vi "BRig_RT__Case_Exp__State_initTrial2__v11.vi"(0 "input_dataCurrent":u16[](array[numeric]), 1 "input_dataTrial":u16[][](array[numeric]), 3 "input_dataExp":u16[](array[numeric]), 6 "input_dataBlock":u16[][](array[numeric]), 8 "input_dataLC":u16[](array[numeric])) -> (7 "output_L_Wrong_Laser_l2":bool, 9 "output_L_Wrong_Event_l2":bool, 10 "output_L_Power_l1":dbl, 11 "output_L_Reward_Laser_l2":bool, 12 "output_L_Power_l2":dbl, 13 "output_L_Reward_Event_l2":bool, 14 "output_dataCurrent":u16[](array[numeric]), 15 "output_dataTrial":u16[][](array[numeric]), 16 "output_L_Reward_Event_l1":bool, 17 "output_L_Reward_Laser_l1":bool, 18 "output_L_Wrong_Event_l1":bool, 19 "output_L_Wrong_Laser_l1":bool)   [LabVIEW 2014]
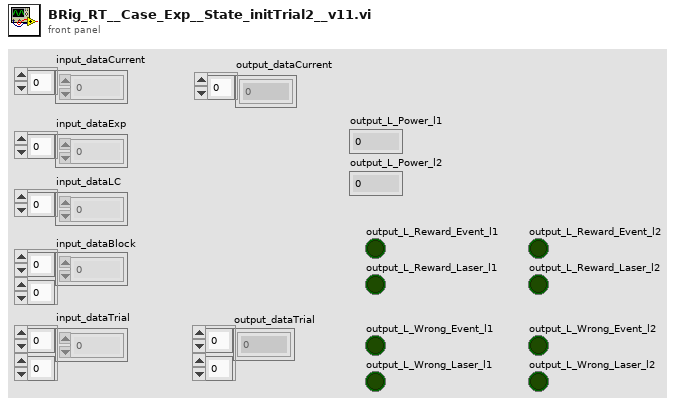
[diagram p1: front panel]
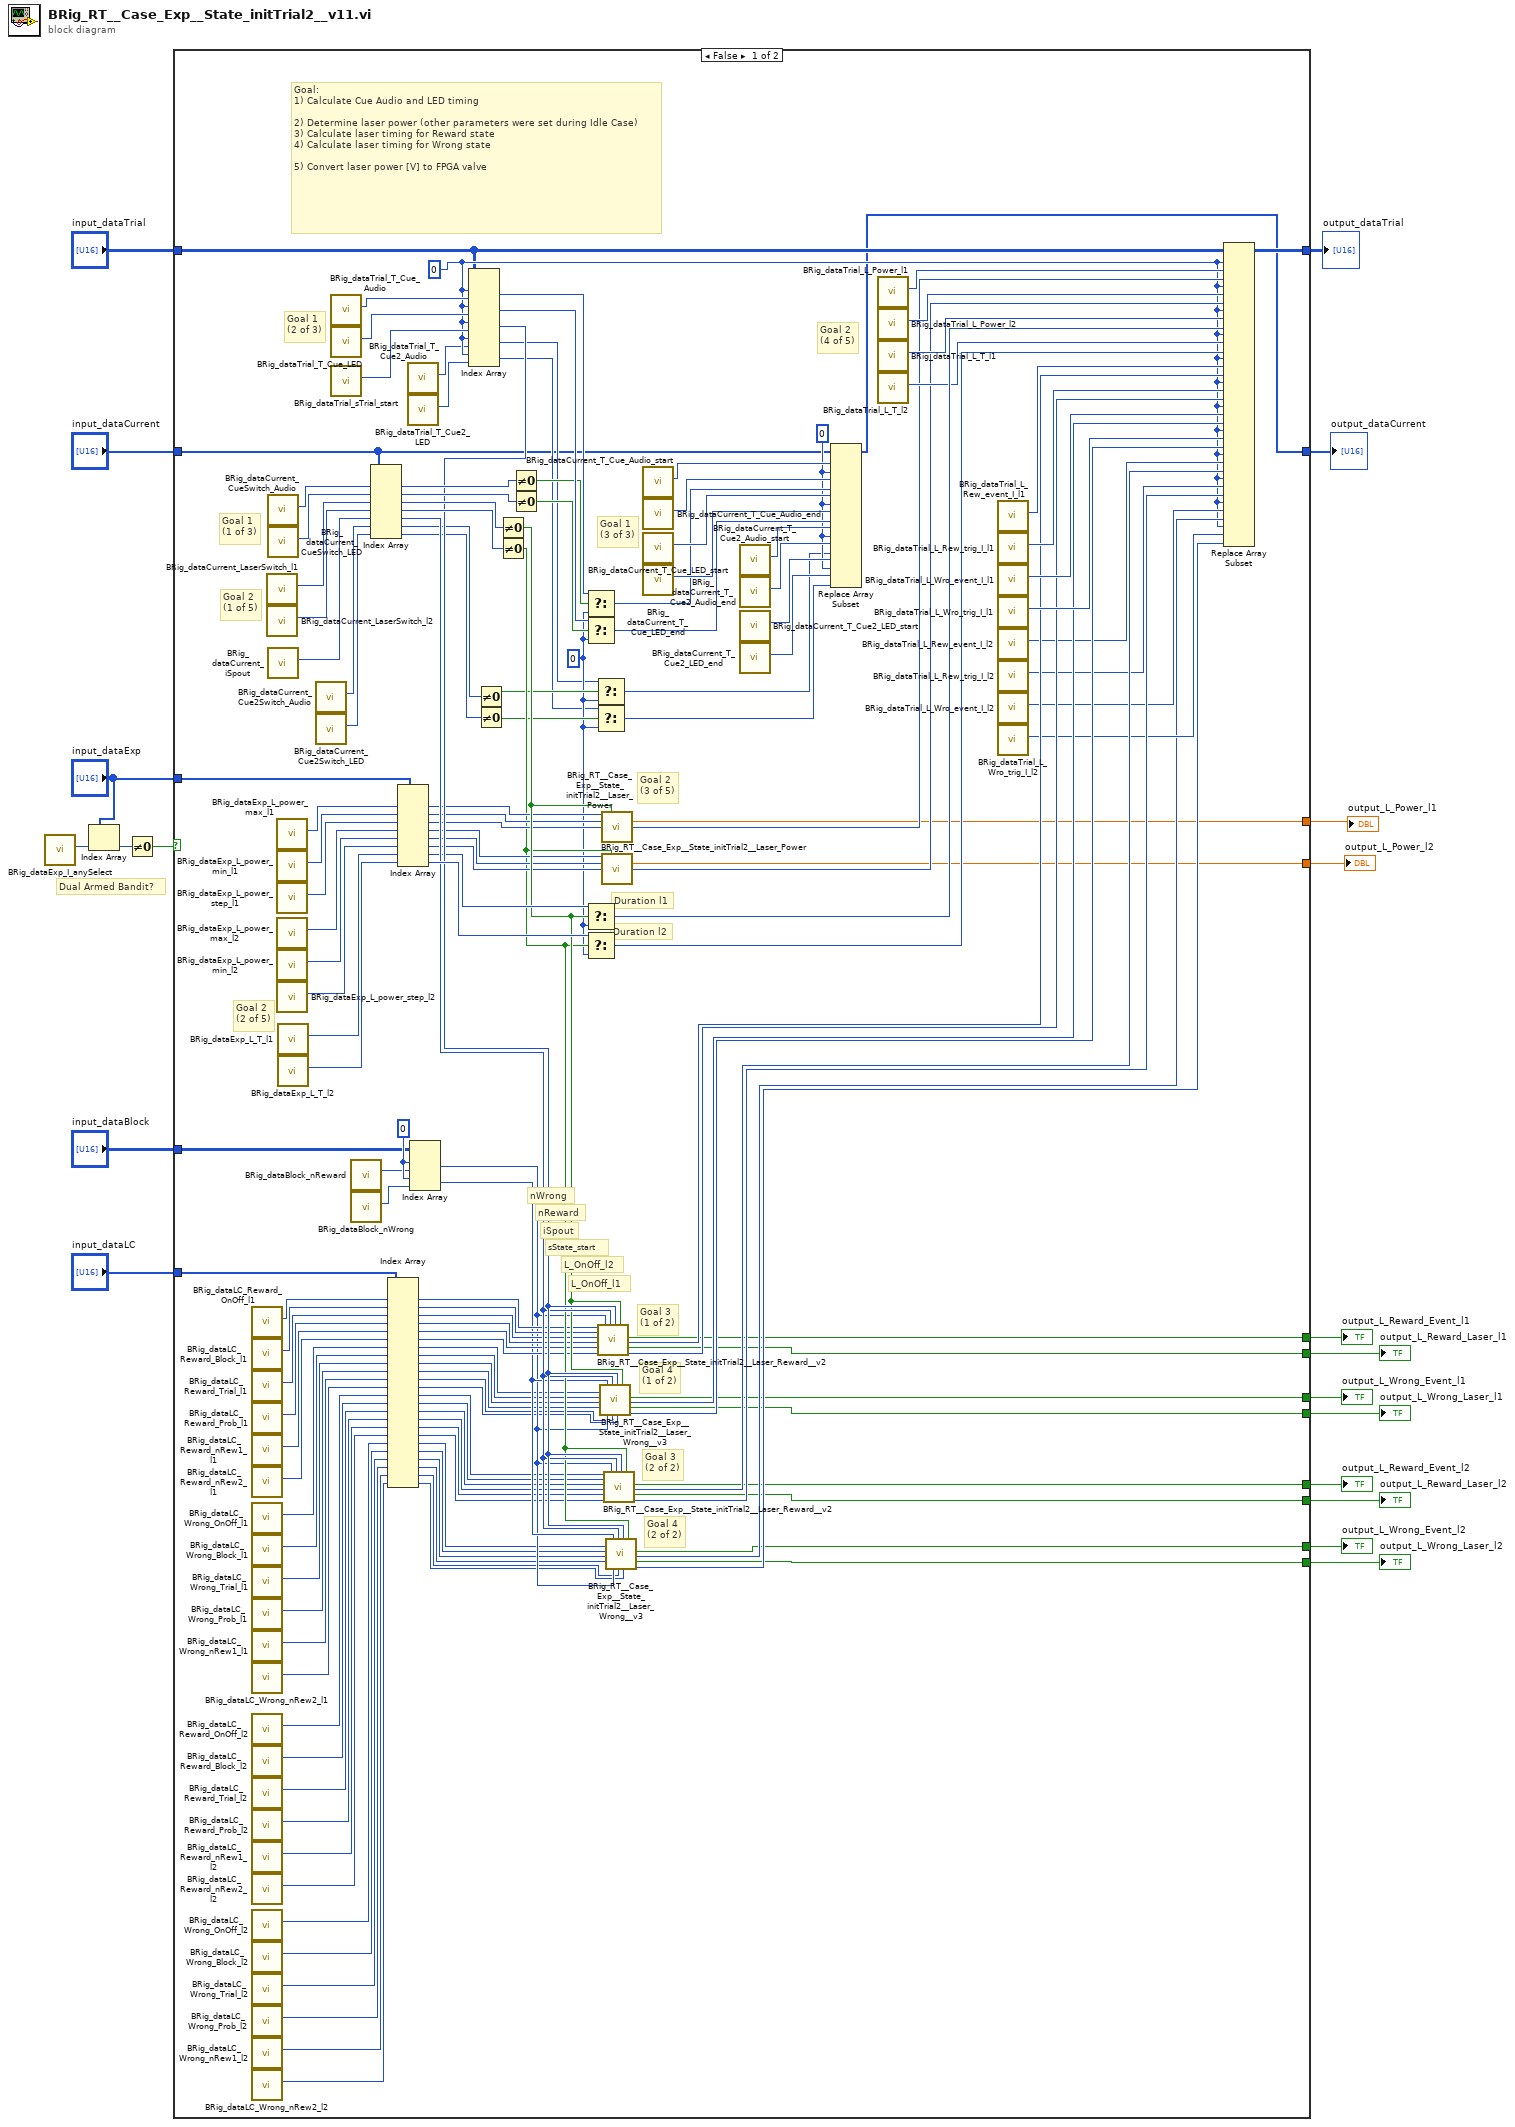
[diagram p0: block diagram]
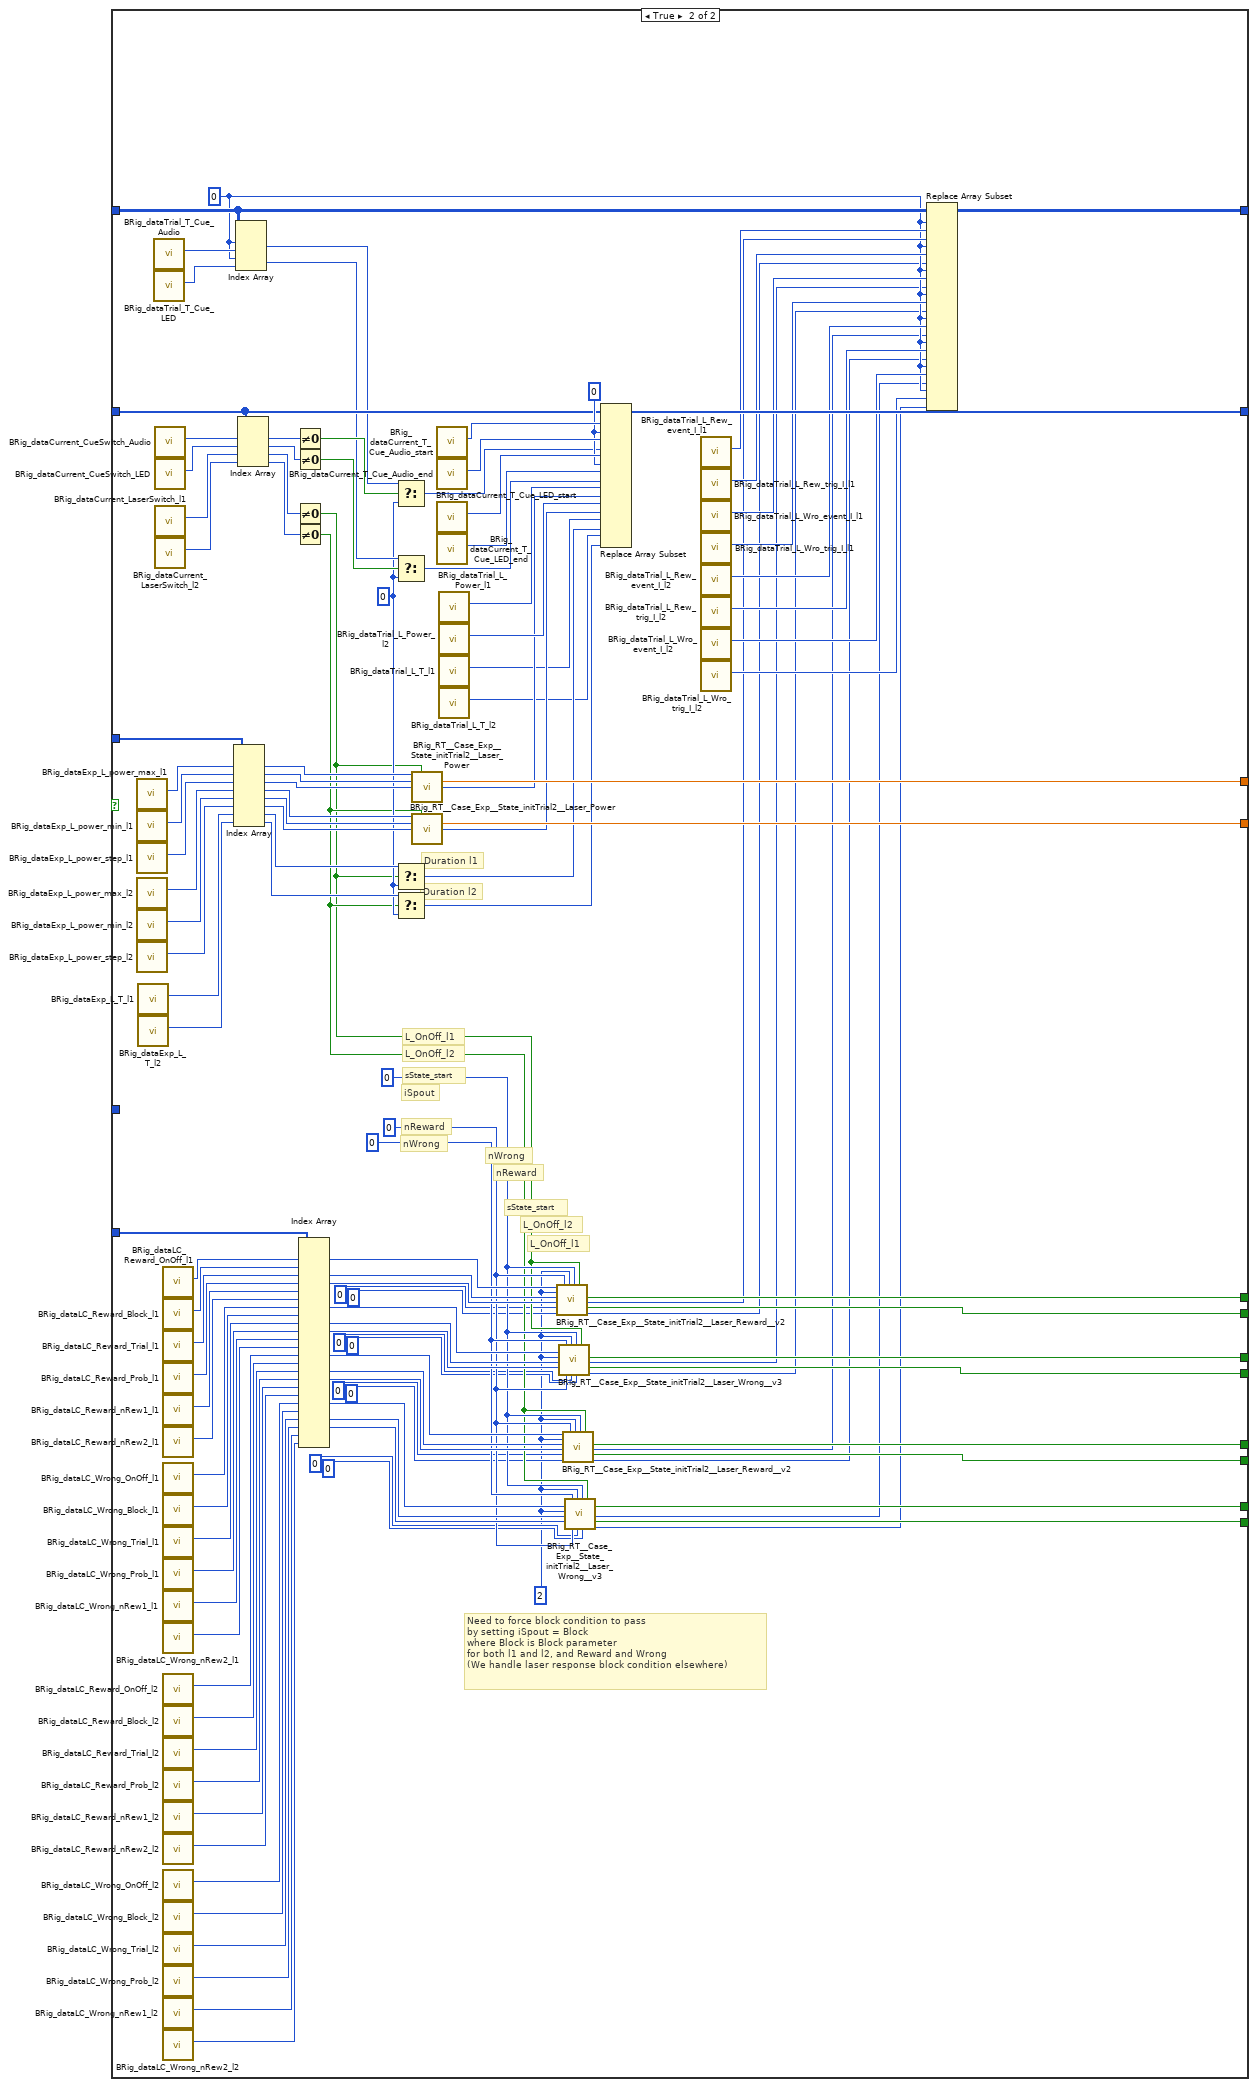
[diagram p2: hidden frame]
diagram:
  # "Dual Armed Bandit?"
  n1 = call "BRig_dataExp_I_anySelect.vi"() -> ("output_I_anySelect"=w5:i32)  [unwired: 11 in]
  n2 = Index Array(array="input_dataExp", index=w5) -> (element=w4:u16)
  n3 = Not Equal To 0?(x=w4) -> (x != 0?=w3:bool)
  n4 = case shown="False" w3 {
    tunnel: [w37 w186] -> w20
    tunnel: "input_dataTrial" -> [w36 w187]
    tunnel: "input_dataCurrent" -> [w35 w289]
    tunnel: "input_dataExp" -> [w34 w265]
    tunnel: "input_dataBlock" -> [w33 _]
    tunnel: "input_dataLC" -> [w32 w225]
    tunnel: [w31 w211] -> w15
    tunnel: [w30 w210] -> w14
    tunnel: [w29 w209] -> w13
    tunnel: [w28 w208] -> w12
    tunnel: [w27 w207] -> w11
    tunnel: [w26 w206] -> w10
    tunnel: [w25 w205] -> w9
    tunnel: [w24 w204] -> w8
    tunnel: [w23 w262] -> w7
    tunnel: [w22 w263] -> w6
    tunnel: [w21 w288] -> w1
    frame False {
      w85 = 0 ("disabled index (row)")
      w105 = 0
      w96 = u16 0 ("f")
      w89 = u16 0 ("new element/subarray")
      # "nWrong"
      # "nReward"
      # "L_OnOff_l2"
      # "Goal 2\n(3 of 5)"
      # "Goal 4\n(2 of 2)"
      # "Goal 4\n(1 of 2)"
      # "Goal 3\n(2 of 2)"
      # "Goal 3\n(1 of 2)"
      # "L_OnOff_l1"
      # "sState_start"
      # "iSpout"
      # "Goal 2\n(4 of 5)"
      # "Goal 2\n(2 of 5)"
      # "Duration l2"
      # "Duration l1"
      # "Goal 2\n(1 of 5)"
      # "Goal 1\n(3 of 3)"
      # "Goal 1\n(2 of 3)"
      # "Goal 1\n(1 of 3)"
      # "Goal:\n1) Calculate Cue Audio and LED timing\n\n2) Determine laser power (other parameters were set during Idle Case)\n3) Calculate laser timing for Reward state\n4) Calculate laser timing for Wrong state\n\n5) Convert laser power [V] to FPGA valve"
      n5 = call "BRig_dataLC_Reward_OnOff_l1.vi"() -> ("output_Reward_OnOff"=w142:i32)  [unwired: 11 in]
      n6 = call "BRig_dataLC_Reward_Block_l1.vi"() -> ("output_Reward_Block"=w141:i32)  [unwired: 11 in]
      n7 = call "BRig_dataLC_Reward_Trial_l1.vi"() -> ("output_Reward_Trial"=w140:i32)  [unwired: 11 in]
      n8 = call "BRig_dataLC_Reward_Prob_l1.vi"() -> ("output_Reward_Prob"=w139:i32)  [unwired: 11 in]
      n9 = call "BRig_dataLC_Reward_nRew1_l1.vi"() -> ("output_Reward_nRew1_l1"=w79:i32)  [unwired: 11 in]
      n10 = call "BRig_dataLC_Reward_nRew2_l1.vi"() -> ("output_Reward_nRew2_l1"=w78:i32)  [unwired: 11 in]
      n11 = call "BRig_dataLC_Wrong_OnOff_l1.vi"() -> ("output_Wrong_OnOff"=w75:i32)  [unwired: 11 in]
      n12 = call "BRig_dataLC_Wrong_Block_l1.vi"() -> ("output_Wrong_Block"=w74:i32)  [unwired: 11 in]
      n13 = call "BRig_dataLC_Wrong_Trial_l1.vi"() -> ("output_Wrong_Trial"=w73:i32)  [unwired: 11 in]
      n14 = call "BRig_dataLC_Wrong_Prob_l1.vi"() -> ("output_Wrong_Prob"=w72:i32)  [unwired: 11 in]
      n15 = call "BRig_dataLC_Wrong_nRew1_l1.vi"() -> ("output_Wrong_nRew1_l1"=w53:i32)  [unwired: 11 in]
      n16 = call "BRig_dataLC_Wrong_nRew2_l1.vi"() -> ("output_Wrong_nRew2_l1"=w52:i32)  [unwired: 11 in]
      n17 = call "BRig_dataLC_Reward_OnOff_l2.vi"() -> ("output_Reward_OnOff_l2"=w60:i32)  [unwired: 11 in]
      n18 = call "BRig_dataLC_Reward_Block_l2.vi"() -> ("output_Reward_Block_l2"=w61:i32)  [unwired: 11 in]
      n19 = call "BRig_dataLC_Reward_Trial_l2.vi"() -> ("output_Reward_Trial_l2"=w62:i32)  [unwired: 11 in]
      n20 = call "BRig_dataLC_Reward_Prob_l2.vi"() -> ("output_Reward_Prob_l2"=w63:i32)  [unwired: 11 in]
      n21 = call "BRig_dataLC_Reward_nRew1_l2.vi"() -> ("output_Reward_nRew1_l2"=w64:i32)  [unwired: 11 in]
      n22 = call "BRig_dataLC_Reward_nRew2_l2.vi"() -> ("output_Reward_nRew2_l2"=w65:i32)  [unwired: 11 in]
      n23 = call "BRig_dataLC_Wrong_OnOff_l2.vi"() -> ("output_Wrong_OnOff_l2"=w66:i32)  [unwired: 11 in]
      n24 = call "BRig_dataLC_Wrong_Block_l2.vi"() -> ("output_Wrong_Block_l2"=w67:i32)  [unwired: 11 in]
      n25 = call "BRig_dataLC_Wrong_Trial_l2.vi"() -> ("output_Wrong_Trial_l2"=w68:i32)  [unwired: 11 in]
      n26 = call "BRig_dataLC_Wrong_Prob_l2.vi"() -> ("output_Wrong_Prob_l2"=w69:i32)  [unwired: 11 in]
      n27 = call "BRig_dataLC_Wrong_nRew1_l2.vi"() -> ("output_Wrong_nRew1_l2"=w45:i32)  [unwired: 11 in]
      n28 = call "BRig_dataLC_Wrong_nRew2_l2.vi"() -> ("output_Wrong_nRew2_l2"=w44:i32)  [unwired: 11 in]
      n29 = call "BRig_dataCurrent_LaserSwitch_l1.vi"() -> ("output_LaserSwitch_l1"=w161:i32)  [unwired: 11 in]
      n30 = call "BRig_dataCurrent_LaserSwitch_l2.vi"() -> ("output_LaserSwitch_l2"=w160:i32)  [unwired: 11 in]
      n31 = call "BRig_dataCurrent_CueSwitch_Audio.vi"() -> ("output_CueSwitch_Audio"=w175:i32)  [unwired: 11 in]
      n32 = call "BRig_dataCurrent_CueSwitch_LED.vi"() -> ("output_CueSwitch_LED"=w174:i32)  [unwired: 11 in]
      n33 = call "BRig_dataCurrent_iSpout.vi"() -> ("output_iSpout"=w136:i32)  [unwired: 11 in]
      n34 = call "BRig_dataExp_L_power_max_l1.vi"() -> ("output_L_power_max_l1"=w159:i32)  [unwired: 11 in]
      n35 = call "BRig_dataExp_L_power_min_l1.vi"() -> ("output_L_power_min_l1"=w158:i32)  [unwired: 11 in]
      n36 = call "BRig_dataExp_L_power_step_l1.vi"() -> ("output_L_power_step_l1"=w157:i32)  [unwired: 11 in]
      n37 = call "BRig_dataExp_L_power_max_l2.vi"() -> ("output_L_power_max_l2"=w156:i32)  [unwired: 11 in]
      n38 = call "BRig_dataExp_L_power_min_l2.vi"() -> ("output_L_power_min_l2"=w155:i32)  [unwired: 11 in]
      n39 = call "BRig_dataExp_L_power_step_l2.vi"() -> ("output_L_power_step_l2"=w154:i32)  [unwired: 11 in]
      n40 = call "BRig_dataExp_L_T_l1.vi"() -> ("output_L_T_l1"=w153:i32)  [unwired: 11 in]
      n41 = call "BRig_dataExp_L_T_l2.vi"() -> ("output_L_T_l2"=w152:i32)  [unwired: 11 in]
      n42 = call "BRig_dataCurrent_Cue2Switch_Audio.vi"() -> ("output_Cue2Switch_Audio"=w102:i32)  [unwired: 11 in]
      n43 = call "BRig_dataCurrent_Cue2Switch_LED.vi"() -> ("output_Cue2Switch_LED"=w101:i32)  [unwired: 11 in]
      n44 = call "BRig_dataTrial_T_Cue_Audio.vi"() -> ("output_T_Cue_Audio"=w166:i32)  [unwired: 11 in]
      n45 = call "BRig_dataTrial_T_Cue_LED.vi"() -> ("output_T_Cue_LED"=w165:i32)  [unwired: 11 in]
      n46 = call "BRig_dataTrial_sTrial_start.vi"() -> ("output_sTrial_start"=w135:i32)  [unwired: 11 in]
      n47 = call "BRig_dataBlock_nReward.vi"() -> ("output_nReward"=w84:i32)  [unwired: 11 in]
      n48 = call "BRig_dataBlock_nWrong.vi"() -> ("output_nWrong"=w86:i32)  [unwired: 11 in]
      n49 = Index Array(array=w35, index #1=w175, index #2=w174, index #3=w161, index #4=w160, index #5=w136, index #6=w102, index #7=w101) -> (element #1=w169:u16, element #2=w168:u16, element #3=w138:u16, element #4=w137:u16, element #5=w133:u16, element #6=w100:u16, element #7=w99:u16)
      n50 = Index Array(array=w32, index #1=w142, index #2=w141, index #3=w140, index #4=w139, index #5=w79, index #6=w78, index #7=w75, index #8=w74, index #9=w73, index #10=w72, index #11=w53, index #12=w52, index #13=w60, index #14=w61, index #15=w62, index #16=w63, index #17=w64, index #18=w65, index #19=w66, index #20=w67, index #21=w68, index #22=w69, index #23=w45, index #24=w44) -> (element #1=w83:u16, element #2=w82:u16, element #3=w81:u16, element #4=w80:u16, element #5=w77:u16, element #6=w76:u16, element #7=w51:u16, element #8=w50:u16, element #9=w49:u16, element #10=w48:u16, element #11=w47:u16, element #12=w46:u16, element #13=w54:u16, element #14=w55:u16, element #15=w56:u16, element #16=w57:u16, element #17=w58:u16, element #18=w59:u16, element #19=w43:u16, element #20=w42:u16, element #21=w41:u16, element #22=w40:u16, element #23=w39:u16, element #24=w38:u16)
      n51 = Index Array(array=w34, index #1=w159, index #2=w158, index #3=w157, index #4=w156, index #5=w155, index #6=w154, index #7=w153, index #8=w152) -> (element #1=w114:u16, element #2=w113:u16, element #3=w112:u16, element #4=w110:u16, element #5=w109:u16, element #6=w108:u16, element #7=w116:u16, element #8=w149:u16)
      n52 = call "BRig_dataTrial_T_Cue2_Audio.vi"() -> ("output_T_Cue2_Audio"=w104:i32)  [unwired: 11 in]
      n53 = call "BRig_dataTrial_T_Cue2_LED.vi"() -> ("output_T_Cue2_LED"=w103:i32)  [unwired: 11 in]
      n54 = Index Array(array=w33, index (row) #1=w85, index (col) #1=w84, index (row) #2=w85, index (col) #2=w86) -> (element #1=w70:u16, element #2=w71:u16)
      n55 = Index Array(array=w36, index (row) #1=w105, index (col) #1=w166, index (row) #2=w105, index (col) #2=w165, index (row) #3=w105, index (col) #3=w135, index (row) #4=w105, index (col) #4=w104, index (row) #5=w105, index (col) #5=w103) -> (element #1=w164:u16, element #2=w163:u16, element #3=w134:u16, element #4=w95:u16, element #5=w94:u16)
      n56 = Not Equal To 0?(x=w100) -> (x != 0?=w98:bool)
      n57 = Not Equal To 0?(x=w99) -> (x != 0?=w97:bool)
      n58 = Not Equal To 0?(x=w138) -> (x != 0?=w115:bool)
      n59 = Not Equal To 0?(x=w137) -> (x != 0?=w107:bool)
      n60 = Not Equal To 0?(x=w169) -> (x != 0?=w151:bool)
      n61 = Not Equal To 0?(x=w168) -> (x != 0?=w150:bool)
      n62 = Select(t=w164, s=w151, f=w96) -> (s? t:f=w167:u16)
      n63 = Select(t=w163, s=w150, f=w96) -> (s? t:f=w162:u16)
      n64 = Select(t=w116, s=w115, f=w96) -> (s? t:f=w145:u16)
      n65 = Select(t=w149, s=w107, f=w96) -> (s? t:f=w143:u16)
      n66 = Select(t=w95, s=w98, f=w96) -> (s? t:f=w88:u16)
      n67 = Select(t=w94, s=w97, f=w96) -> (s? t:f=w87:u16)
      n68 = call "BRig_RT__Case_Exp__State_initTrial2__Laser_Reward__v2.vi"("input_L_OnOff"=w83, "input_L_Block"=w82, "input_L_Trial"=w81, "input_L_Probability"=w80, "input_L_nRew1"=w77, "input_L_nRew2"=w76, "input_nReward"=w70, "input_iSpout"=w133, "input_sState_start"=w134, "input_LaserSwitch"=w115) -> ("output_LR_Event"=w31:bool, "output_LR_Event_num"=w128:u16, "output_LR_Laser"=w30:bool, "output_LR_Laser_num"=w127:u16)  [unwired: 6 in]
      n69 = call "BRig_RT__Case_Exp__State_initTrial2__Laser_Wrong__v3.vi"("input_L_OnOff"=w51, "input_L_Block"=w50, "input_L_Trial"=w49, "input_L_Probability"=w48, "input_nWrong"=w71, "input_nReward"=w70, "input_iSpout"=w133, "input_L_nRew1"=w47, "input_sState_start"=w134, "input_L_nRew2"=w46, "input_LaserSwitch"=w115) -> ("output_LR_Event"=w29:bool, "output_LR_Event_num"=w126:u16, "output_LR_Laser"=w28:bool, "output_LR_Laser_num"=w125:u16)  [unwired: 5 in]
      n70 = call "BRig_RT__Case_Exp__State_initTrial2__Laser_Power.vi"("input_L_Power_max__x100"=w114, "input_LaserSwitch"=w115, "input_L_Power_min__x100"=w113, "input_L_Power_step__x100"=w112) -> ("output_L_Power"=w22:dbl, "output_L_Power_x100"=w111:u16)  [unwired: 10 in]
      n71 = call "BRig_RT__Case_Exp__State_initTrial2__Laser_Power.vi"("input_L_Power_max__x100"=w110, "input_LaserSwitch"=w107, "input_L_Power_min__x100"=w109, "input_L_Power_step__x100"=w108) -> ("output_L_Power"=w23:dbl, "output_L_Power_x100"=w106:u16)  [unwired: 10 in]
      n72 = call "BRig_RT__Case_Exp__State_initTrial2__Laser_Reward__v2.vi"("input_L_OnOff"=w54, "input_L_Block"=w55, "input_L_Trial"=w56, "input_L_Probability"=w57, "input_L_nRew1"=w58, "input_L_nRew2"=w59, "input_nReward"=w70, "input_iSpout"=w133, "input_sState_start"=w134, "input_LaserSwitch"=w107) -> ("output_LR_Event"=w27:bool, "output_LR_Event_num"=w123:u16, "output_LR_Laser"=w26:bool, "output_LR_Laser_num"=w121:u16)  [unwired: 6 in]
      n73 = call "BRig_RT__Case_Exp__State_initTrial2__Laser_Wrong__v3.vi"("input_L_OnOff"=w43, "input_L_Block"=w42, "input_L_Trial"=w41, "input_L_Probability"=w40, "input_nWrong"=w71, "input_nReward"=w70, "input_iSpout"=w133, "input_L_nRew1"=w39, "input_sState_start"=w134, "input_L_nRew2"=w38, "input_LaserSwitch"=w107) -> ("output_LR_Event"=w25:bool, "output_LR_Event_num"=w118:u16, "output_LR_Laser"=w24:bool, "output_LR_Laser_num"=w117:u16)  [unwired: 5 in]
      n74 = call "BRig_dataCurrent_T_Cue_Audio_start.vi"() -> ("output_T_Cue_Audio_start"=w173:i32)  [unwired: 11 in]
      n75 = call "BRig_dataCurrent_T_Cue_Audio_end.vi"() -> ("output_T_Cue_Audio_end"=w172:i32)  [unwired: 11 in]
      n76 = call "BRig_dataCurrent_T_Cue_LED_start.vi"() -> ("output_T_Cue_LED_start"=w171:i32)  [unwired: 11 in]
      n77 = call "BRig_dataCurrent_T_Cue_LED_end.vi"() -> ("output_T_Cue_LED_end"=w170:i32)  [unwired: 11 in]
      n78 = call "BRig_dataCurrent_T_Cue2_Audio_start.vi"() -> ("output_T_Cue2_Audio_start"=w93:i32)  [unwired: 11 in]
      n79 = call "BRig_dataCurrent_T_Cue2_Audio_end.vi"() -> ("output_T_Cue2_Audio_end"=w92:i32)  [unwired: 11 in]
      n80 = call "BRig_dataCurrent_T_Cue2_LED_start.vi"() -> ("output_T_Cue2_LED_start"=w91:i32)  [unwired: 11 in]
      n81 = call "BRig_dataCurrent_T_Cue2_LED_end.vi"() -> ("output_T_Cue2_LED_end"=w90:i32)  [unwired: 11 in]
      n82 = Replace Array Subset(array=w35, new element #1=w89, index #1=w173, new element #2=w167, index #2=w172, new element #3=w89, index #3=w171, new element #4=w162, index #4=w170, new element #5=w89, index #5=w93, new element #6=w88, index #6=w92, new element #7=w89, index #7=w91, new element #8=w87, index #8=w90) -> (w21:u16[])
      n83 = call "BRig_dataTrial_L_Power_l1.vi"() -> ("output_L_Power_l1"=w148:i32)  [unwired: 11 in]
      n84 = call "BRig_dataTrial_L_Power_l2.vi"() -> ("output_L_Power_l2"=w147:i32)  [unwired: 11 in]
      n85 = call "BRig_dataTrial_L_T_l1.vi"() -> ("output_L_T_l1"=w146:i32)  [unwired: 11 in]
      n86 = call "BRig_dataTrial_L_T_l2.vi"() -> ("output_L_T_l2"=w144:i32)  [unwired: 11 in]
      n87 = call "BRig_dataTrial_L_Rew_event_I_l1.vi"() -> ("output_L_Rew_event_I_l1"=w132:i32)  [unwired: 11 in]
      n88 = call "BRig_dataTrial_L_Rew_trig_I_l1.vi"() -> ("output_L_Rew_trig_I_l1"=w131:i32)  [unwired: 11 in]
      n89 = call "BRig_dataTrial_L_Wro_event_I_l1.vi"() -> ("output_L_Wro_event_I_l1"=w130:i32)  [unwired: 11 in]
      n90 = call "BRig_dataTrial_L_Wro_trig_I_l1.vi"() -> ("output_L_Wro_trig_I_l1"=w129:i32)  [unwired: 11 in]
      n91 = call "BRig_dataTrial_L_Rew_event_I_l2.vi"() -> ("output_L_Rew_event_I_l2"=w124:i32)  [unwired: 11 in]
      n92 = call "BRig_dataTrial_L_Rew_trig_I_l2.vi"() -> ("output_L_Rew_trig_I_l2"=w122:i32)  [unwired: 11 in]
      n93 = call "BRig_dataTrial_L_Wro_event_I_l2.vi"() -> ("output_L_Wro_event_I_l2"=w120:i32)  [unwired: 11 in]
      n94 = call "BRig_dataTrial_L_Wro_trig_I_l2.vi"() -> ("output_L_Wro_trig_I_l2"=w119:i32)  [unwired: 11 in]
      n95 = Replace Array Subset(array=w36, new element #1=w111, index (row) #1=w105, index (col) #1=w148, new element #2=w106, index (row) #2=w105, index (col) #2=w147, new element #3=w145, index (row) #3=w105, index (col) #3=w146, new element #4=w143, index (row) #4=w105, index (col) #4=w144, new element #5=w128, index (row) #5=w105, index (col) #5=w132, new element #6=w127, index (row) #6=w105, index (col) #6=w131, new element #7=w126, index (row) #7=w105, index (col) #7=w130, new element #8=w125, index (row) #8=w105, index (col) #8=w129, new element #9=w123, index (row) #9=w105, index (col) #9=w124, new element #10=w121, index (row) #10=w105, index (col) #10=w122, new element #11=w118, index (row) #11=w105, index (col) #11=w120, new element #12=w117, index (row) #12=w105, index (col) #12=w119) -> (w37:u16[][])
    }
    frame True {
      w176 = u16 2 ("input_sState_start")
      w222 = u16 0 ("disabled index (row)")
      w223 = u16 0 ("disabled index (row)")
      w224 = u16 0 ("disabled index (row)")
      w264 = u16 0 ("f")
      w290 = u16 0 ("new element/subarray")
      w184 = 0
      # "Need to force block condition to pass\nby setting iSpout = Block\nwhere Block is Block parameter\nfor both l1 and l2, and Reward and Wrong\n(We handle laser response block condition elsewhere)"
      # "L_OnOff_l1"
      # "L_OnOff_l2"
      # "sState_start"
      # "iSpout"
      # "nReward"
      # "nWrong"
      # "nWrong"
      # "nReward"
      # "L_OnOff_l2"
      # "L_OnOff_l1"
      # "sState_start"
      # "Duration l2"
      # "Duration l1"
      n96 = call "BRig_dataExp_L_power_max_l1.vi"() -> ("output_L_power_max_l1"=w281:i32)  [unwired: 11 in]
      n97 = call "BRig_dataExp_L_power_min_l1.vi"() -> ("output_L_power_min_l1"=w280:i32)  [unwired: 11 in]
      n98 = call "BRig_dataExp_L_power_step_l1.vi"() -> ("output_L_power_step_l1"=w279:i32)  [unwired: 11 in]
      n99 = call "BRig_dataExp_L_power_max_l2.vi"() -> ("output_L_power_max_l2"=w278:i32)  [unwired: 11 in]
      n100 = call "BRig_dataExp_L_power_min_l2.vi"() -> ("output_L_power_min_l2"=w277:i32)  [unwired: 11 in]
      n101 = call "BRig_dataExp_L_power_step_l2.vi"() -> ("output_L_power_step_l2"=w276:i32)  [unwired: 11 in]
      n102 = call "BRig_dataExp_L_T_l1.vi"() -> ("output_L_T_l1"=w275:i32)  [unwired: 11 in]
      n103 = call "BRig_dataExp_L_T_l2.vi"() -> ("output_L_T_l2"=w274:i32)  [unwired: 11 in]
      n104 = call "BRig_dataTrial_T_Cue_Audio.vi"() -> ("output_T_Cue_Audio"=w304:i32)  [unwired: 11 in]
      n105 = call "BRig_dataTrial_T_Cue_LED.vi"() -> ("output_T_Cue_LED"=w303:i32)  [unwired: 11 in]
      n106 = call "BRig_dataCurrent_CueSwitch_Audio.vi"() -> ("output_CueSwitch_Audio"=w302:i32)  [unwired: 11 in]
      n107 = call "BRig_dataCurrent_CueSwitch_LED.vi"() -> ("output_CueSwitch_LED"=w301:i32)  [unwired: 11 in]
      n108 = call "BRig_dataCurrent_LaserSwitch_l1.vi"() -> ("output_LaserSwitch_l1"=w300:i32)  [unwired: 11 in]
      n109 = call "BRig_dataCurrent_LaserSwitch_l2.vi"() -> ("output_LaserSwitch_l2"=w299:i32)  [unwired: 11 in]
      n110 = call "BRig_dataLC_Reward_OnOff_l1.vi"() -> ("output_Reward_OnOff"=w261:i32)  [unwired: 11 in]
      n111 = call "BRig_dataLC_Reward_Block_l1.vi"() -> ("output_Reward_Block"=w260:i32)  [unwired: 11 in]
      n112 = call "BRig_dataLC_Reward_Trial_l1.vi"() -> ("output_Reward_Trial"=w259:i32)  [unwired: 11 in]
      n113 = call "BRig_dataLC_Reward_Prob_l1.vi"() -> ("output_Reward_Prob"=w258:i32)  [unwired: 11 in]
      n114 = call "BRig_dataLC_Reward_nRew1_l1.vi"() -> ("output_Reward_nRew1_l1"=w254:i32)  [unwired: 11 in]
      n115 = call "BRig_dataLC_Reward_nRew2_l1.vi"() -> ("output_Reward_nRew2_l1"=w253:i32)  [unwired: 11 in]
      n116 = call "BRig_dataLC_Wrong_OnOff_l1.vi"() -> ("output_Wrong_OnOff"=w252:i32)  [unwired: 11 in]
      n117 = call "BRig_dataLC_Wrong_Block_l1.vi"() -> ("output_Wrong_Block"=w251:i32)  [unwired: 11 in]
      n118 = call "BRig_dataLC_Wrong_Trial_l1.vi"() -> ("output_Wrong_Trial"=w250:i32)  [unwired: 11 in]
      n119 = call "BRig_dataLC_Wrong_Prob_l1.vi"() -> ("output_Wrong_Prob"=w249:i32)  [unwired: 11 in]
      n120 = call "BRig_dataLC_Wrong_nRew1_l1.vi"() -> ("output_Wrong_nRew1_l1"=w235:i32)  [unwired: 11 in]
      n121 = call "BRig_dataLC_Wrong_nRew2_l1.vi"() -> ("output_Wrong_nRew2_l1"=w234:i32)  [unwired: 11 in]
      n122 = call "BRig_dataLC_Reward_OnOff_l2.vi"() -> ("output_Reward_OnOff_l2"=w239:i32)  [unwired: 11 in]
      n123 = call "BRig_dataLC_Reward_Block_l2.vi"() -> ("output_Reward_Block_l2"=w240:i32)  [unwired: 11 in]
      n124 = call "BRig_dataLC_Reward_Trial_l2.vi"() -> ("output_Reward_Trial_l2"=w241:i32)  [unwired: 11 in]
      n125 = call "BRig_dataLC_Reward_Prob_l2.vi"() -> ("output_Reward_Prob_l2"=w242:i32)  [unwired: 11 in]
      n126 = call "BRig_dataLC_Reward_nRew1_l2.vi"() -> ("output_Reward_nRew1_l2"=w243:i32)  [unwired: 11 in]
      n127 = call "BRig_dataLC_Reward_nRew2_l2.vi"() -> ("output_Reward_nRew2_l2"=w244:i32)  [unwired: 11 in]
      n128 = call "BRig_dataLC_Wrong_OnOff_l2.vi"() -> ("output_Wrong_OnOff_l2"=w245:i32)  [unwired: 11 in]
      n129 = call "BRig_dataLC_Wrong_Block_l2.vi"() -> ("output_Wrong_Block_l2"=w246:i32)  [unwired: 11 in]
      n130 = call "BRig_dataLC_Wrong_Trial_l2.vi"() -> ("output_Wrong_Trial_l2"=w247:i32)  [unwired: 11 in]
      n131 = call "BRig_dataLC_Wrong_Prob_l2.vi"() -> ("output_Wrong_Prob_l2"=w248:i32)  [unwired: 11 in]
      n132 = call "BRig_dataLC_Wrong_nRew1_l2.vi"() -> ("output_Wrong_nRew1_l2"=w230:i32)  [unwired: 11 in]
      n133 = call "BRig_dataLC_Wrong_nRew2_l2.vi"() -> ("output_Wrong_nRew2_l2"=w229:i32)  [unwired: 11 in]
      n134 = Index Array(array=w265, index #1=w281, index #2=w280, index #3=w279, index #4=w278, index #5=w277, index #6=w276, index #7=w275, index #8=w274) -> (element #1=w271:u16, element #2=w270:u16, element #3=w269:u16, element #4=w268:u16, element #5=w267:u16, element #6=w266:u16, element #7=w272:u16, element #8=w273:u16)
      n135 = Index Array(array=w187, index (row) #1=w184, index (col) #1=w304, index (row) #2=w184, index (col) #2=w303) -> (element #1=w285:u16, element #2=w284:u16)
      n136 = Index Array(array=w289, index #1=w302, index #2=w301, index #3=w300, index #4=w299) -> (element #1=w298:u16, element #2=w297:u16, element #3=w296:u16, element #4=w295:u16)
      n137 = Not Equal To 0?(x=w298) -> (x != 0?=w287:bool)
      n138 = Not Equal To 0?(x=w297) -> (x != 0?=w286:bool)
      n139 = Not Equal To 0?(x=w296) -> (x != 0?=w220:bool)
      n140 = Not Equal To 0?(x=w295) -> (x != 0?=w221:bool)
      n141 = Index Array(array=w225, index #1=w261, index #2=w260, index #3=w259, index #4=w258, index #5=w254, index #6=w253, index #7=w252, index #8=w251, index #9=w250, index #10=w249, index #11=w235, index #12=w234, index #13=w239, index #14=w240, index #15=w241, index #16=w242, index #17=w243, index #18=w244, index #19=w245, index #20=w246, index #21=w247, index #22=w248, index #23=w230, index #24=w229) -> (element #1=w257:u16, element #3=w256:u16, element #4=w255:u16, element #7=w233:u16, element #9=w232:u16, element #10=w231:u16, element #13=w236:u16, element #15=w237:u16, element #16=w238:u16, element #19=w228:u16, element #21=w227:u16, element #22=w226:u16)  [unwired: 12 out]
      n142 = Select(t=w285, s=w287, f=w264) -> (s? t:f=w283:u16)
      n143 = Select(t=w284, s=w286, f=w264) -> (s? t:f=w282:u16)
      n144 = Select(t=w272, s=w220, f=w264) -> (s? t:f=w198:u16)
      n145 = Select(t=w273, s=w221, f=w264) -> (s? t:f=w196:u16)
      n146 = call "BRig_RT__Case_Exp__State_initTrial2__Laser_Power.vi"("input_L_Power_max__x100"=w271, "input_LaserSwitch"=w220, "input_L_Power_min__x100"=w270, "input_L_Power_step__x100"=w269) -> ("output_L_Power"=w263:dbl, "output_L_Power_x100"=w201:u16)  [unwired: 10 in]
      n147 = call "BRig_RT__Case_Exp__State_initTrial2__Laser_Power.vi"("input_L_Power_max__x100"=w268, "input_LaserSwitch"=w221, "input_L_Power_min__x100"=w267, "input_L_Power_step__x100"=w266) -> ("output_L_Power"=w262:dbl, "output_L_Power_x100"=w200:u16)  [unwired: 10 in]
      n148 = call "BRig_dataCurrent_T_Cue_Audio_start.vi"() -> ("output_T_Cue_Audio_start"=w294:i32)  [unwired: 11 in]
      n149 = call "BRig_dataCurrent_T_Cue_Audio_end.vi"() -> ("output_T_Cue_Audio_end"=w293:i32)  [unwired: 11 in]
      n150 = call "BRig_dataCurrent_T_Cue_LED_start.vi"() -> ("output_T_Cue_LED_start"=w292:i32)  [unwired: 11 in]
      n151 = call "BRig_dataCurrent_T_Cue_LED_end.vi"() -> ("output_T_Cue_LED_end"=w291:i32)  [unwired: 11 in]
      n152 = call "BRig_dataTrial_L_Power_l1.vi"() -> ("output_L_Power_l1"=w203:i32)  [unwired: 11 in]
      n153 = call "BRig_dataTrial_L_Power_l2.vi"() -> ("output_L_Power_l2"=w202:i32)  [unwired: 11 in]
      n154 = call "BRig_dataTrial_L_T_l1.vi"() -> ("output_L_T_l1"=w199:i32)  [unwired: 11 in]
      n155 = call "BRig_dataTrial_L_T_l2.vi"() -> ("output_L_T_l2"=w197:i32)  [unwired: 11 in]
      n156 = call "BRig_RT__Case_Exp__State_initTrial2__Laser_Reward__v2.vi"("input_L_OnOff"=w257, "input_L_Block"=w176, "input_L_Trial"=w256, "input_L_Probability"=w255, "input_L_nRew1"=u16 0 ("disabled index (row)"), "input_L_nRew2"=u16 0 ("disabled index (row)"), "input_nReward"=w223, "input_iSpout"=w176, "input_sState_start"=w222, "input_LaserSwitch"=w220) -> ("output_LR_Event"=w211:bool, "output_LR_Event_num"=w185:u16, "output_LR_Laser"=w210:bool, "output_LR_Laser_num"=w183:u16)  [unwired: 6 in]
      n157 = call "BRig_RT__Case_Exp__State_initTrial2__Laser_Wrong__v3.vi"("input_L_OnOff"=w233, "input_L_Block"=w176, "input_L_Trial"=w232, "input_L_Probability"=w231, "input_nWrong"=w224, "input_nReward"=w223, "input_iSpout"=w176, "input_L_nRew1"=u16 0 ("disabled index (row)"), "input_sState_start"=w222, "input_L_nRew2"=u16 0 ("disabled index (row)"), "input_LaserSwitch"=w220) -> ("output_LR_Event"=w209:bool, "output_LR_Event_num"=w182:u16, "output_LR_Laser"=w208:bool, "output_LR_Laser_num"=w181:u16)  [unwired: 5 in]
      n158 = call "BRig_RT__Case_Exp__State_initTrial2__Laser_Reward__v2.vi"("input_L_OnOff"=w236, "input_L_Block"=w176, "input_L_Trial"=w237, "input_L_Probability"=w238, "input_L_nRew1"=u16 0 ("disabled index (row)"), "input_L_nRew2"=u16 0 ("disabled index (row)"), "input_nReward"=w223, "input_iSpout"=w176, "input_sState_start"=w222, "input_LaserSwitch"=w221) -> ("output_LR_Event"=w207:bool, "output_LR_Event_num"=w180:u16, "output_LR_Laser"=w206:bool, "output_LR_Laser_num"=w179:u16)  [unwired: 6 in]
      n159 = call "BRig_RT__Case_Exp__State_initTrial2__Laser_Wrong__v3.vi"("input_L_OnOff"=w228, "input_L_Block"=w176, "input_L_Trial"=w227, "input_L_Probability"=w226, "input_nWrong"=w224, "input_nReward"=w223, "input_iSpout"=w176, "input_L_nRew1"=u16 0 ("disabled index (row)"), "input_sState_start"=w222, "input_L_nRew2"=u16 0 ("disabled index (row)"), "input_LaserSwitch"=w221) -> ("output_LR_Event"=w205:bool, "output_LR_Event_num"=w178:u16, "output_LR_Laser"=w204:bool, "output_LR_Laser_num"=w177:u16)  [unwired: 5 in]
      n160 = Replace Array Subset(array=w289, new element #1=w290, index #1=w294, new element #2=w283, index #2=w293, new element #3=w290, index #3=w292, new element #4=w282, index #4=w291, new element #5=w201, index #5=w203, new element #6=w200, index #6=w202, new element #7=w198, index #7=w199, new element #8=w196, index #8=w197) -> (w288:u16[])
      n161 = call "BRig_dataTrial_L_Rew_event_I_l1.vi"() -> ("output_L_Rew_event_I_l1"=w195:i32)  [unwired: 11 in]
      n162 = call "BRig_dataTrial_L_Rew_trig_I_l1.vi"() -> ("output_L_Rew_trig_I_l1"=w194:i32)  [unwired: 11 in]
      n163 = call "BRig_dataTrial_L_Wro_event_I_l1.vi"() -> ("output_L_Wro_event_I_l1"=w193:i32)  [unwired: 11 in]
      n164 = call "BRig_dataTrial_L_Wro_trig_I_l1.vi"() -> ("output_L_Wro_trig_I_l1"=w192:i32)  [unwired: 11 in]
      n165 = call "BRig_dataTrial_L_Rew_event_I_l2.vi"() -> ("output_L_Rew_event_I_l2"=w191:i32)  [unwired: 11 in]
      n166 = call "BRig_dataTrial_L_Rew_trig_I_l2.vi"() -> ("output_L_Rew_trig_I_l2"=w190:i32)  [unwired: 11 in]
      n167 = call "BRig_dataTrial_L_Wro_event_I_l2.vi"() -> ("output_L_Wro_event_I_l2"=w189:i32)  [unwired: 11 in]
      n168 = call "BRig_dataTrial_L_Wro_trig_I_l2.vi"() -> ("output_L_Wro_trig_I_l2"=w188:i32)  [unwired: 11 in]
      n169 = Replace Array Subset(array=w187, new element #1=w185, index (row) #1=w184, index (col) #1=w195, new element #2=w183, index (row) #2=w184, index (col) #2=w194, new element #3=w182, index (row) #3=w184, index (col) #3=w193, new element #4=w181, index (row) #4=w184, index (col) #4=w192, new element #5=w180, index (row) #5=w184, index (col) #5=w191, new element #6=w179, index (row) #6=w184, index (col) #6=w190, new element #7=w178, index (row) #7=w184, index (col) #7=w189, new element #8=w177, index (row) #8=w184, index (col) #8=w188) -> (w186:u16[][])
    }
  }
  "output_dataTrial" <- w20
  "output_L_Reward_Event_l1" <- w15
  "output_L_Wrong_Event_l1" <- w13
  "output_L_Reward_Event_l2" <- w11
  "output_L_Wrong_Event_l2" <- w9
  "output_L_Reward_Laser_l1" <- w14
  "output_L_Wrong_Laser_l1" <- w12
  "output_L_Reward_Laser_l2" <- w10
  "output_L_Wrong_Laser_l2" <- w8
  "output_L_Power_l2" <- w7
  "output_L_Power_l1" <- w6
  "output_dataCurrent" <- w1
